vi "(Incomplete) Beta Function.vi"   [LabVIEW 2012, in "NI_Gmath.lvlib"]
doc: "Evaluates the beta function or the incomplete beta function. You must manually select the polymorphic instance you want to use."
uses:
  NI_Gmath.lvlib
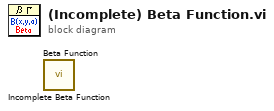
[diagram p0: block diagram]
diagram:
  n1 = call "Incomplete Beta Function.vi"() -> ()  [unwired: 11 in, 1 out]
  n2 = call "Beta Function.vi"() -> ()  [unwired: 11 in, 1 out]
